vi "Read Device Identification Response.vi"(8 "error in (no error)":errorcluster, 10 "Modbus data unit in":refnum<class "Modbus Data Unit (PDU).lvclass">) -> (0 "error out":errorcluster, 2 "objects":cluster{"object ID":u8, "value":string}[](array[cluster]) {"object ID" format="%x"}, 4 "next object ID":u8, 5 "conformity level":u8(ring) items=["None"=0, "Basic Stream"=1, "Regular Stream"=2, "Extended Stream"=3, "Basic Stream/Individual"=129, "Regular Stream/Individual"=130, "Extended Stream/Individual"=131], 6 "done?":bool)   [LabVIEW 2020, in "SubVIs.lvlib" / "Master Function Definition.lvlib"]
uses:
  <vilib>/Modbus/subvis/Data and Functions/Master Function Definition/Master Function Definition.lvlib
  <vilib>/Modbus/subvis/Modbus Data Unit (PDU)/Modbus Data Unit (PDU).lvclass
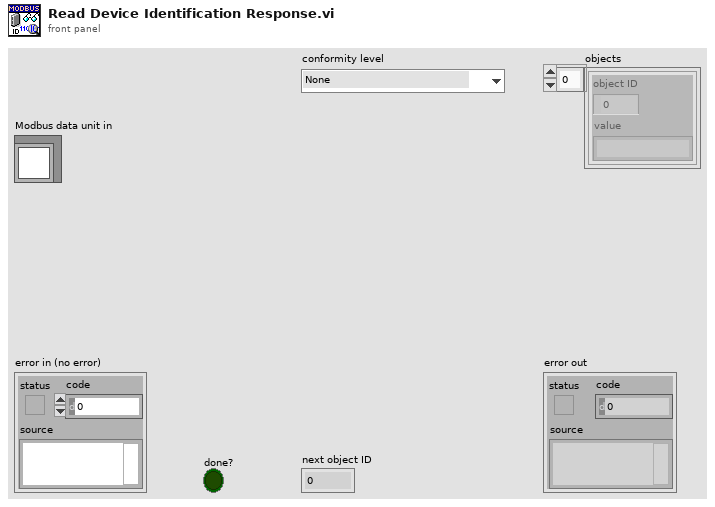
[diagram p1: front panel]
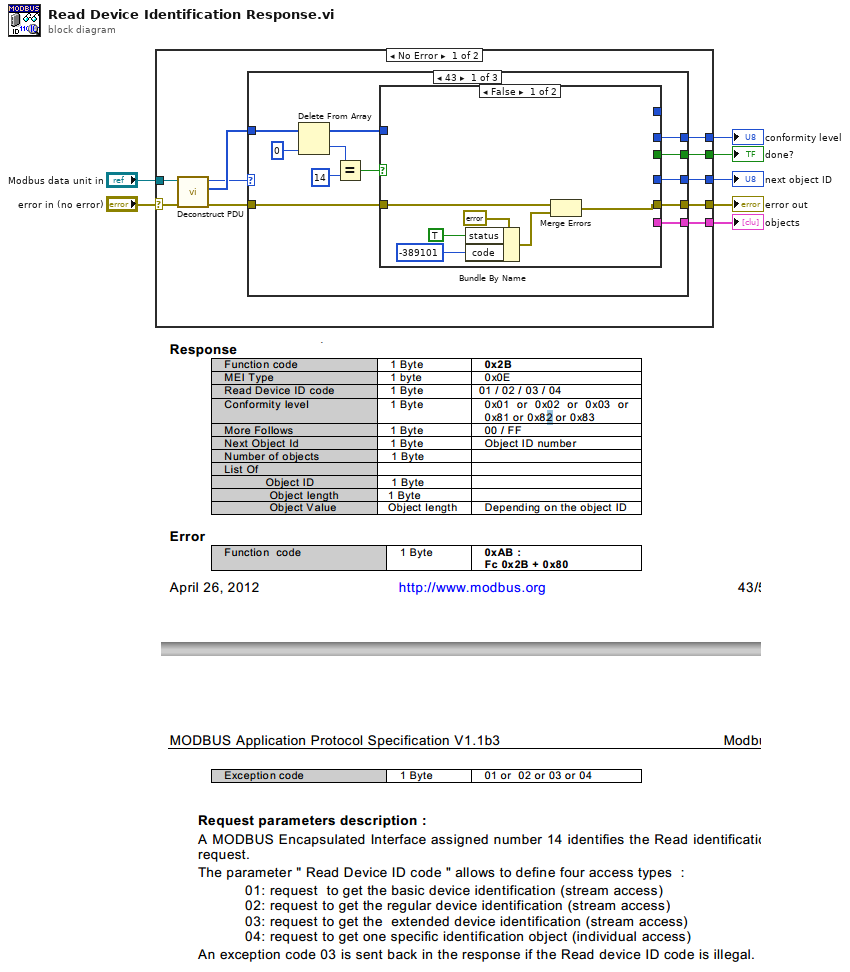
[diagram p0: block diagram]
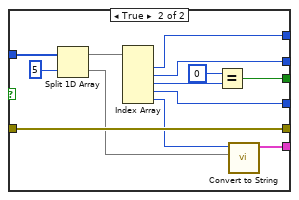
[diagram p2: hidden frame]
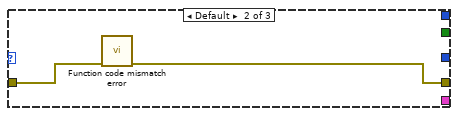
[diagram p3: hidden frame]
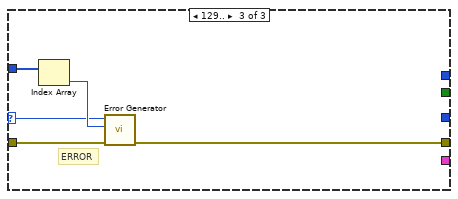
[diagram p4: hidden frame]
diagram:
  n1 = case shown="No Error" "error in (no error)" {
    selector: "error in (no error)" -> [w16 w56]
    tunnel: [w17 w56] -> w6
    tunnel: "Modbus data unit in" -> [w14 _]
    tunnel: [w12 _] -> w3
    tunnel: [w11 _] -> w4
    tunnel: [w10 _] -> w2
    tunnel: [w9 _] -> w1
    frame No Error {
      n2 = call <vilib>:"Deconstruct PDU.vi"("error in (no error)"=w16, "Modbus data unit in"=w14) -> ("error out"=w13:errorcluster, "data"=w15:u8[], "function"=w8:u8)  [unwired: 7 in]
      n3 = case shown="43" w8 {
        selector: w8 -> [_ _ w51]
        tunnel: w13 -> [w27 w50 w52]
        tunnel: w15 -> [w29 _ w55]
        tunnel: [w28 w49 w54] -> w17
        tunnel: [w26 _ _] -> w12
        tunnel: [w25 _ _] -> w11
        tunnel: [w24 _ _] -> w10
        tunnel: [w23 _ _] -> w9
        frame 43 {
          n4 = Delete From Array(array=w29, index=0) -> (deleted portion=w21:u8, array with subset deleted=w22:u8[])  [unwired: 1 in]
          n5 = Equal?(x=w21, y=u8 14) -> (x = y?=w19:bool)
          n6 = case shown="False" w19 {
            tunnel: [_ w39] -> w26
            tunnel: [_ w46] -> w25
            tunnel: [_ w45] -> w24
            tunnel: [_ w44] -> w23
            tunnel: w22 -> [_ w43]
            tunnel: w27 -> [w30 w42]
            tunnel: [w31 w42] -> w28
            tunnel: [_ w36] -> _
            frame False {
              n7 = Bundle By Name(cluster=errorcluster {"status"=FALSE, "code"=0, "source"=""} ("error constant"), "status"=TRUE, "code"=-389101) -> (w34:errorcluster)
              n8 = Merge Errors(w30, w34) -> (w31:errorcluster)
            }
            frame True {
              n9 = Split 1D Array(array=w43, index=5) -> (first subarray=w47:u8[], second subarray=w38:u8[])
              n10 = Index Array(array=w47) -> (element #1=w36:u8, element #2=w46:u8, element #3=w41:u8, element #4=w45:u8, element #5=w37:u8)  [unwired: 5 in]
              n11 = Equal?(x=u8 0, y=w41) -> (x = y?=w39:bool)
              n12 = call <vilib>:"Convert to String.vi"("byte array"=w38, "number of objects"=w37) -> ("objects"=w44:cluster{"object ID":u8, "value":string}[])  [unwired: 9 in]
            }
          }
        }
        frame Default {
          n13 = call <vilib>:"Function code mismatch error.vi"("error in (no error)"=w50) -> ("error out"=w49:errorcluster)  [unwired: 10 in]
        }
        frame 129.. {
          # "ERROR"
          n14 = Index Array(array=w55) -> (element=w53:u8)  [unwired: 1 in]
          n15 = call <vilib>:"Error Generator.vi"("error in (no error)"=w52, "data return (error code)"=w53, "function return"=w51) -> ("error out"=w54:errorcluster)  [unwired: 8 in]
        }
      }
    }
    frame Error {
    }
  }
  "error out" <- w6
  "conformity level" <- w4
  "done?" <- w3
  "next object ID" <- w2
  "objects" <- w1
